vi "Cleanup Conversion Sessions.vi"(10 "DIDs":T1[](array[typedef]) {"Signals"."Byte Order" items=["Little Endian", "Big Endian"]; "Signals"."Data Type" items=["Signed", "Unsigned", "IEEE Float"]}, 11 "DID Lookup":variant) -> (0 "Array":errorcluster[](array[cluster]))   [LabVIEW 2015, in "Diagnostics Addon Engine.lvlib"]
uses:
  Diagnostics Addon Engine.lvlib
  Shared/Types/Frame Parameters.ctl
  Shared/Types/Signal Parameters.ctl
  Shared/SubVIs/GUID Lookup.vi
  Shared/Diagnostics Addon Shared.lvlib
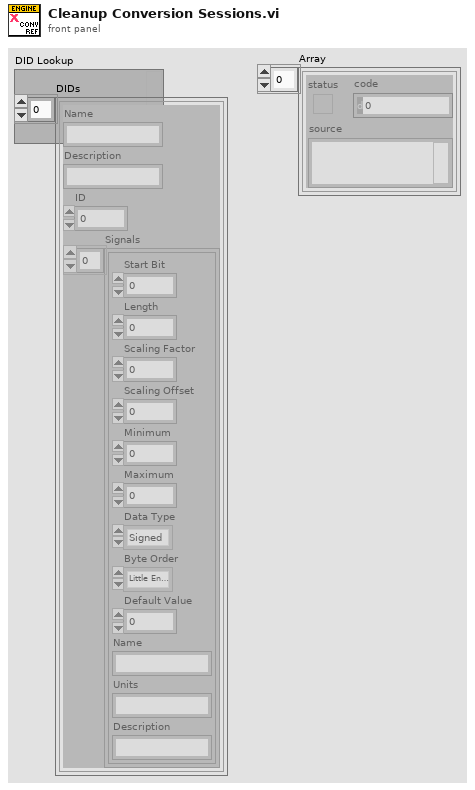
[diagram p1: front panel]
types:
  T1 = typedef "Diagnostics Addon Shared.lvlib/Frame Parameters.ctl" = cluster{"Name":string, "Description":string, "ID":u32, "Signals":T2[]}
  T2 = typedef "Diagnostics Addon Shared.lvlib/Signal Parameters.ctl" = cluster{"Start Bit":u8, "Length":u8, "Scaling Factor":dbl, "Scaling Offset":dbl, "Minimum":dbl, "Maximum":dbl, "Data Type":u32, "Byte Order":u32, "Default Value":dbl, "Name":string, "Units":string, "Description":string}
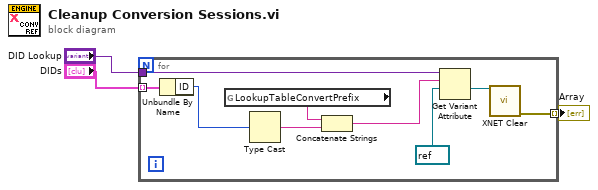
[diagram p0: block diagram]
diagram:
  n1 = for {
    tunnel: [w12] -> w1 mode=indexing
    tunnel: "DIDs" -> [w11] mode=indexing
    tunnel: "DID Lookup" -> [w5]
    n2 = Unbundle By Name(w11) -> ("ID"=w6:u32)
    n3 = global read "GUID Lookup.vi" "LookupTableConvertPrefix"() -> (w8:string)
    n4 = Type Cast(x=w6) -> (*(type *) &x=w7:string)  [unwired: 1 in]
    n5 = Concatenate Strings(w8, w7) -> (w9:string)
    n6 = Get Variant Attribute(Variant=w5, name=w9, default value (empty Variant)=refnum<k21> refnum ("DID Conversion")) -> (value=w4:refnum<k21>)  [unwired: 1 in, 3 out]
    n7 = call <vilib>:"XNET Clear.vi"("session in"=w4) -> ("error out"=w12:errorcluster)  [unwired: 14 in]
  }
  "Array" <- w1
